vi "emi_Time offset holder.vi"(1 "Action(GET)":enum16{"GET", "SET"}(ring), 7 "Offset in":dbl) -> (8 "Offset out":dbl)   [LabVIEW 2011]
doc: "Holder for teh offset time that may be in the emi get time with err"
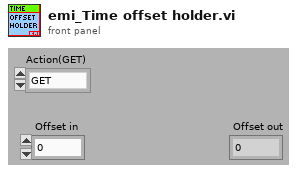
[diagram p1: front panel]
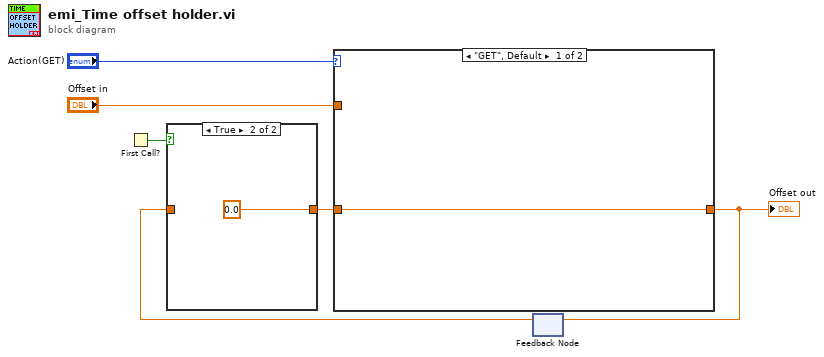
[diagram p0: block diagram]
diagram:
  n1 = First Call?() -> (First Call?: T/F=w4:bool)
  n2 = feedback #1() -> (w5:dbl)  [unwired: 1 in]
  n3 = case shown="True" w4 {
    tunnel: w5 -> [w7 _]
    tunnel: [w7 0.0 ("Offset")] -> w2
    frame False {
    }
    frame True {
    }
  }
  n4 = case shown="\"GET\", Default" "Action(GET)" {
    tunnel: [w9 w10] -> w3
    tunnel: w2 -> [w9 _]
    tunnel: "Offset in" -> [_ w10]
    frame "GET", Default {
    }
    frame "SET" {
    }
  }
  "Offset out" <- w3
  n5 = feedback-in #1(w3) -> ()
